vi "Error Insert_v4.vi"(5 "show call chain? (False)":bool, 6 "error in (no error)":errorcluster, 8 "error message (\"\")":string, 9 "error code (0)":i32) -> (0 "error out":errorcluster)   [LabVIEW 2013]
doc: "Converts an error or warning code to an error cluster. This VI is useful when you receive a return value from a DLL call or when you return user-defined error codes."
uses:
  <vilib>/Utility/error.llb/whitespace.ctl
panel:
  in  "call chain header":string="\n<b>Complete call chain:</b>"
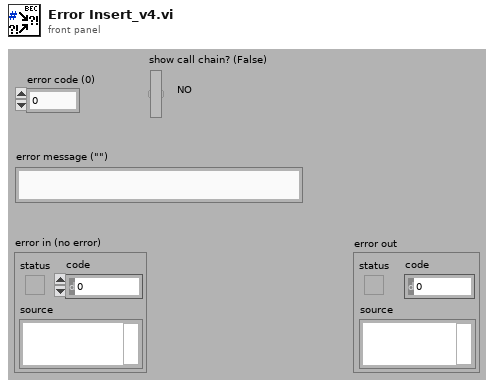
[diagram p1: front panel]
types:
  T1 = typedef "whitespace.ctl" = u16
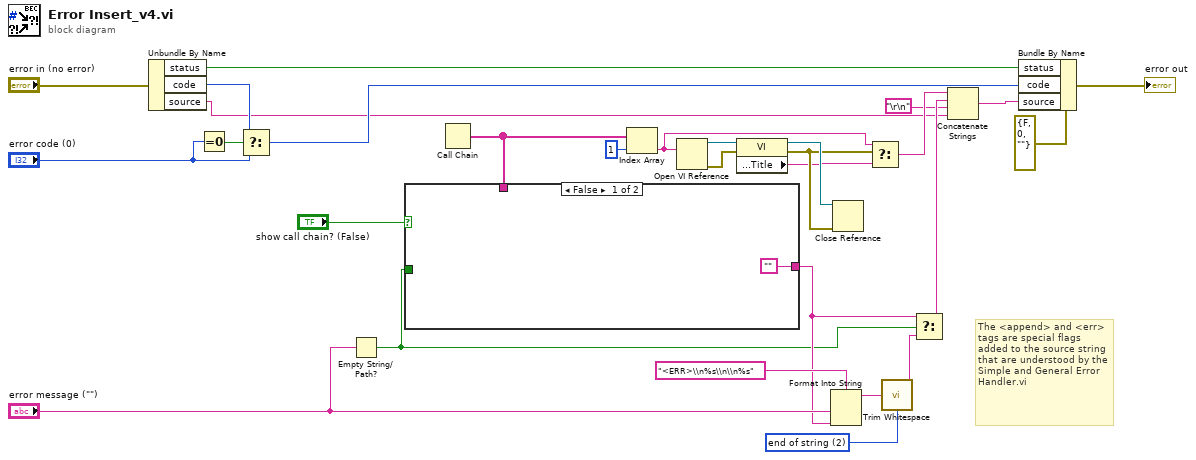
[diagram p0: block diagram]
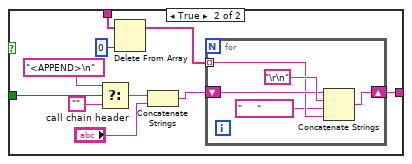
[diagram p2: hidden frame]
diagram:
  w8 = T1 2 items=["both", "start of string", "end of string"] ("location (both)")
  # "The <append> and <err> tags are special flags added to the source string that are understood by the Simple and General Error Handler.vi"
  n1 = Unbundle By Name("error in (no error)") -> ("status"=w3:bool, "code"=w7:i32, "source"=w2:string)
  n2 = Equal To 0?(x="error code (0)") -> (x = 0?=w5:bool)
  n3 = Select(t=w7, s=w5, f="error code (0)") -> (s? t:f=w6:i32)
  n4 = Empty String/Path?(string/path="error message (\"\")") -> (empty?=w11:bool)
  n5 = Call Chain() -> (call chain=w20:string[])
  n6 = case shown="False" "show call chain? (False)" {
    tunnel: ["" w40] -> w13
    tunnel: w20 -> [_ w38]
    tunnel: w11 -> [_ w34]
    frame False {
    }
    frame True {
      n7 = Select(t="<APPEND>\n", s=w34, f="") -> (s? t:f=w31:string)
      n8 = Delete From Array(array=w38, index=0) -> (array with subset deleted=w37:string[])  [unwired: 1 in, 1 out]
      n9 = Concatenate Strings(w31, "call chain header") -> (w35:string)
      n10 = for {
        tunnel: w37 -> [w42] mode=indexing
        shift-right: [w45] -> w40
        shift-left: w35 -> [w43]
        n11 = Concatenate Strings(w43, "\r\n", "     ", w42) -> (w45:string)
      }
    }
  }
  n12 = Index Array(array=w20, index=1) -> (element=w18:string)
  n13 = Open VI Reference(vi path=w18) -> (vi reference=w23:refnum<vi>, error out=w22:errorcluster)  [unwired: 1 in, 4 out]
  n14 = property class="VI"(reference=w23, error in=w22) -> (reference out=w21:refnum<vi>, error out=w19:errorcluster, "Front Panel Window:Title"=w17:string)
  n15 = Format Into String(format string="<ERR>\\n%s\\n\\n%s", "error message (\"\")", w13) -> (resulting string=w10:string)  [unwired: 2 in, 1 out]
  n16 = Close Reference(reference=w21, error in (no error)=w19) -> ()  [unwired: 1 out]
  n17 = Select(t=w18, s=w19, f=w17) -> (s? t:f=w16:string)
  n18 = call <vilib>:"Trim Whitespace.vi"("string"=w10, "location (both)"=w8) -> ("trimmed string"=w9:string)
  n19 = Select(t=w13, s=w11, f=w9) -> (s? t:f=w12:string)
  n20 = Concatenate Strings(w16, w12, "\r\n", w2) -> (w25:string)
  n21 = Bundle By Name(cluster=errorcluster {"status"=FALSE, "code"=0, "source"=""} ("error out"), "status"=w3, "code"=w6, "source"=w25) -> (→"error out":errorcluster)
